vi "Close Command.vi"(0 "command":refnum<k21>, 11 "error in (no error)":errorcluster) -> (15 "error out":errorcluster)   [LabVIEW 2020, in "SLSC.lvlib"]
doc: "Closes an open reference to an SLSC command."
uses:
  <vilib>/SLSC/SLSC.lvlib
  nislsclvapi.dll
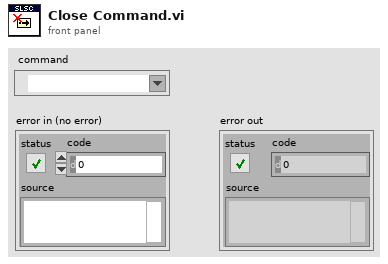
[diagram p1: front panel]
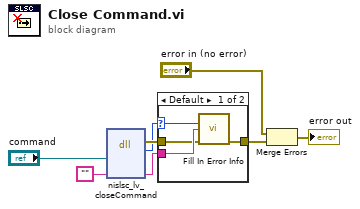
[diagram p0: block diagram]
diagram:
  n1 = dll-call lib="nislsclvapi.*" fn="nislsc_lv_closeCommand"("commandRefObj"="command", "extendedErrorInfo"="") -> (error out=w7:errorcluster, "return type"=w6:i32, "extendedErrorInfo"=w8:string)  [unwired: 6 in, 1 out]
  n2 = case shown="Default" w6 {
    selector: w6 -> [w12 _]
    tunnel: w8 -> [w11 _]
    tunnel: w7 -> [w10 w13]
    tunnel: [w9 w13] -> w2
    frame Default {
      n3 = call <vilib>:"Fill In Error Info.vi"("status code"=w12, "extended error info"=w11, "error in"=w10) -> ("error out"=w9:errorcluster)  [unwired: 12 in]
    }
    frame 0 {
    }
  }
  n4 = Merge Errors("error in (no error)", w2) -> (→"error out":errorcluster)
